vi "Windows Get CPU Loads.vi"(7 "Action":enum16{"init", "read", "cleanup"}(ring), 8 "error in (no error)":errorcluster) -> (0 "error out":errorcluster, 2 "CPU Loads":dbl[](array[numeric]), 3 "# of CPUs":u32)   [LabVIEW 2020, in "Telemetry Engine.lvlib"]
doc: "This FGV uses .net Performance Counters to read each CPU core load present in the Windows system."
uses:
  Telemetry Engine.lvlib
  90b97e59-b598-4dd5-8027-b7fd49914e4d.vi
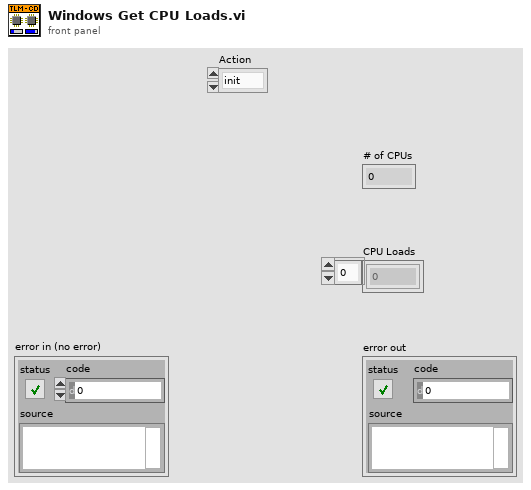
[diagram p1: front panel]
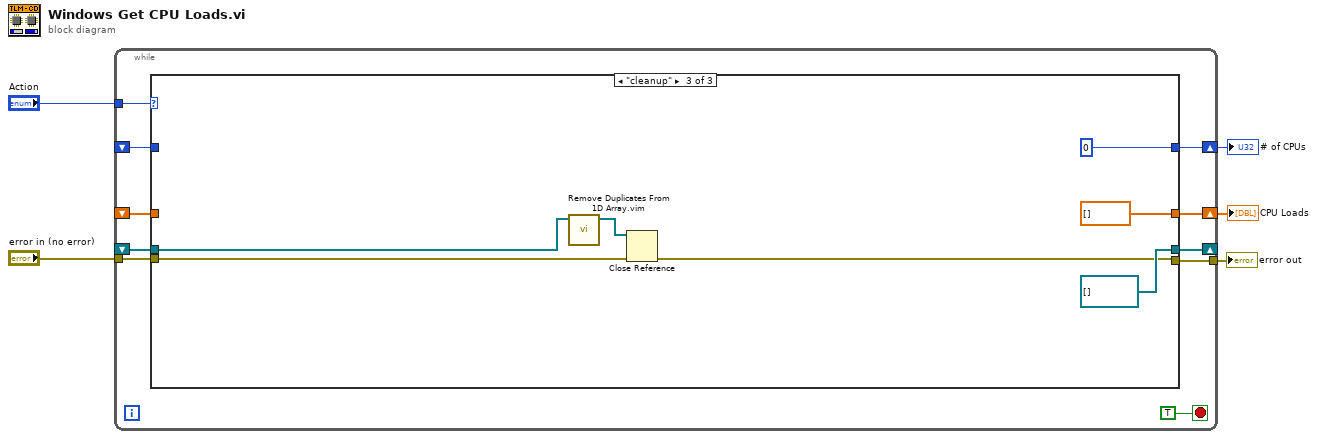
[diagram p0: block diagram]
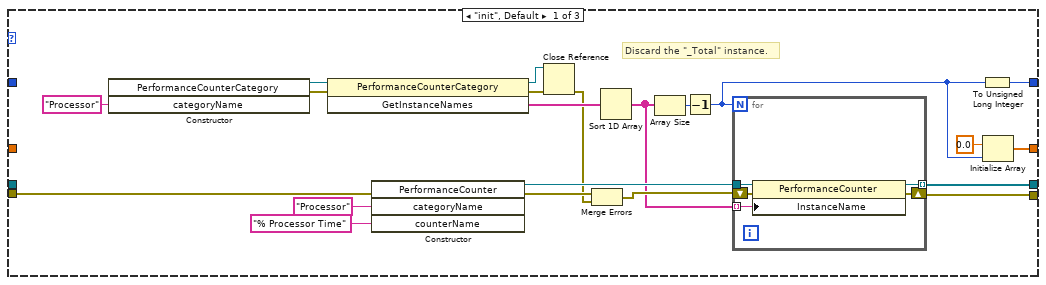
[diagram p2: hidden frame]
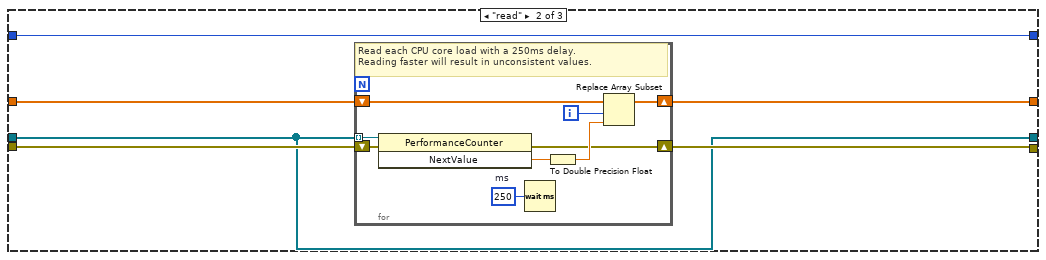
[diagram p3: hidden frame]
diagram:
  n1 = while {
    tunnel: "Action" -> [w14]
    shift-right: [w13] -> w3
    shift-left: _ -> [w12]
    tunnel: "error in (no error)" -> [w11]
    shift-right: [w10] -> _
    shift-left: _ -> [w9]
    tunnel: [w7] -> w1
    shift-right: [w8] -> w2
    shift-left: _ -> [w6]
    stop <- TRUE stop-if-true
    n2 = case shown="\"cleanup\"" w14 {
      tunnel: [w17 w47 u32 0] -> w13
      tunnel: w12 -> [_ w47 _]
      tunnel: w11 -> [w22 w45 w61]
      tunnel: [w21 w42 refnum<k24>[] []] -> w10
      tunnel: w9 -> [_ w42 w57]
      tunnel: [w19 w46 dbl[] []] -> w8
      tunnel: [w20 w44 w60] -> w7
      tunnel: w6 -> [_ w43 _]
      frame "init", Default {
        # "Discard the \"_Total\" instance."
        n3 = constructor class="PerformanceCounterCategory"("categoryName"="Processor") -> (reference out=w35:refnum<k24>, error out=w25:errorcluster)  [unwired: 3 in, 2 out]
        n4 = invoke class="PerformanceCounterCategory" method="GetInstanceNames"(reference=w35, error in=w25) -> (reference out=w28:refnum<k24>, error out=w27:errorcluster, "GetInstanceNames"=w34:string[])  [unwired: 1 in]
        n5 = constructor class="PerformanceCounter"(error in=w22, "categoryName"="Processor", "counterName"="% Processor Time") -> (reference out=w31:refnum<k24>, error out=w30:errorcluster)  [unwired: 2 in, 3 out]
        n6 = Close Reference(reference=w28, error in (no error)=w27) -> (error out=w26:errorcluster)
        n7 = Merge Errors(w30, w26) -> (w29:errorcluster)
        n8 = Sort 1D Array(array=w34) -> (sorted array=w23:string[])
        n9 = Array Size(array=w23) -> (size(s)=w24:i32)
        n10 = Decrement(x=w24) -> (x-1=w16:i32)
        n11 = for {
          N: w16 -> [_]
          tunnel: w31 -> [w41]
          tunnel: [w39] -> w21 mode=indexing
          shift-right: [w38] -> w20
          shift-left: w29 -> [w40]
          tunnel: w23 -> [w37] mode=indexing
          n12 = property class="PerformanceCounter"(reference=w41, error in=w40, "InstanceName"=w37) -> (reference out=w39:refnum<k24>, error out=w38:errorcluster)
        }
        n13 = To Unsigned Long Integer(number=w16) -> (unsigned 32bit integer=w17:u32)
        n14 = Initialize Array(0.0 ("element"), w16) -> (w19:dbl[])
      }
      frame "read" {
        n15 = for {
          shift-right: [w49] -> w44
          shift-left: w45 -> [w55]
          tunnel: w42 -> [w56] mode=indexing
          shift-right: [w53] -> w46
          shift-left: w43 -> [w52]
          i -> [w54]
          w48 = u32 250  # ms
          # "Read each CPU core load with a 250ms delay.\nReading faster will result in unconsistent values."
          n16 = invoke class="PerformanceCounter" method="NextValue"(reference=w56, error in=w55) -> (error out=w49:errorcluster, "NextValue"=w51:sgl)  [unwired: 1 in, 1 out]
          n17 = Wait (ms)(milliseconds to wait=w48) -> ()  [unwired: 1 out]
          n18 = To Double Precision Float(number=w51) -> (double precision float=w50:dbl)
          n19 = Replace Array Subset(array=w52, new element=w50, index=w54) -> (w53:dbl[])
        }
      }
      frame "cleanup" {
        n20 = call "Remove Duplicates From 1D Array.vim"("array"=w57) -> ("array with duplicates removed"=w58:refnum<k24>[])  [unwired: 10 in]
        n21 = Close Reference(reference=w58, error in (no error)=w61) -> (error out=w60:errorcluster)
      }
    }
  }
  "# of CPUs" <- w3
  "CPU Loads" <- w2
  "error out" <- w1
